vi "npks.vi"() -> ()   [LabVIEW 2015]
uses:
  <vilib>/LabVIEW Open Source Project/MQTT Control Packets/Control Packets/SUBACK/Subscription Success Code.ctl
  <vilib>/LabVIEW Open Source Project/MQTT Control Packets/Control Packets/ControlPacket/QualityOfService -- enum.ctl
  <vilib>/LabVIEW Open Source Project/MQTT Control Packets/Control Packets/SUBSCRIBE/Topic Subscription -- cluster.ctl
  <vilib>/LabVIEW Open Source Project/MQTT Control Packets/Control Packets/CONNECT/ConnectFlags -- cluster.ctl
  <vilib>/LabVIEW Open Source Project/MQTT Client/Client class/Client.lvclass/Client.ctl
  <vilib>/LabVIEW Open Source Project/MQTT Connection/MQTT_Base/Base Class/MQTT_Base.lvclass/MQTT_Base.ctl
  <vilib>/LabVIEW Open Source Project/MQTT Control Packets/Control Packets/ControlPacket/ControlPacket.lvclass/ControlPacket.ctl
  <vilib>/Modbus/master/Create Master Instance (Serial).vi
  <vilib>/LabVIEW Open Source Project/MQTT Control Packets/Control Packets/PUBLISH/PUBLISH.lvclass
  <vilib>/Modbus/master/Modbus Master.lvclass
  <vilib>/LabVIEW Open Source Project/MQTT Client/Client class/Client.lvclass
  <vilib>/LabVIEW Open Source Project/MQTT Connection/MQTT_Base/Base Class/MQTT_Base.lvclass
  <vilib>/LabVIEW Open Source Project/MQTT Control Packets/Control Packets/ControlPacket/ControlPacket.lvclass
  <vilib>/LabVIEW Open Source Project/Connection/Connection.TCP/Connection.TCP.lvclass
  <vilib>/LabVIEW Open Source Project/Connection/Connection.LocalQueue/Connection.LocalQueue.lvclass
  <vilib>/LabVIEW Open Source Project/Connection/Connection/Connection.lvclass
  <vilib>/LabVIEW Open Source Project/MQTT Control Packets/Control Packets/SUBACK/SUBACK.lvclass
  <vilib>/LabVIEW Open Source Project/MQTT Control Packets/Control Packets/SUBSCRIBE/SUBSCRIBE.lvclass
  <vilib>/LabVIEW Open Source Project/MQTT Control Packets/Control Packets/CONNECT/CONNECT.lvclass
panel:
  out "K":bool
  in  "Payload":T1={"Will Topic"="", "Will Message"="", "Username"="jCpxJWfzRMyJc3yBgeDZF8tX4bProa3f", "Password"="dyi3Gar4LryWnGSwkNjPS2jYQKdPeLnd"}
  in  "Will Message":string
  in  "Will Topic":string
  out "N":bool
  out "P":bool
  in  "SET POINT N":dbl=300.0
  in  "SET POINT K":dbl=20.0
  in  "holding register value K":u16
  in  "SET POINT P":dbl=300.0
  in  "holding register value P":u16
  out "error out 9":errorcluster
  out "K":string="                        199"
  out "Type 3":variant
  out "Topic 3":string
  out "error out 8":cluster{}
  out "Suback":bool
  out "source 2":string
  out "code":i32
  out "status":bool
  out "source":string
  in  "error in (no error)":errorcluster
  in  "ID (empty:generate new)":string="e22b6e7b-a166-44ae-bd9e-56b8868e9341"
  in  "Connect Flags":T2={"Reserved"=FALSE, "Clean Session"=TRUE, "Will Flag"=FALSE, "Will QoS 1"=FALSE, "Will QoS 2"=FALSE, "Will Retain"=FALSE, "Password Flag"=TRUE, "User Name Flag"=TRUE}
  out "error out 7":errorcluster
  out "error out 2":errorcluster
  out "Incoming Message":u8[](array[numeric]) format="%08b"
  out "error out 6":errorcluster
  out "P":string
  out "Type 2":variant
  out "Topic 2":string
  out "error out 5":cluster{}
  out "error out 4":errorcluster
  out "N":string
  out "Type":variant
  out "Topic":string
  out "error out 3":cluster{"status":bool, "code":i32}
  in  "Subscribe":bool
  in  "Topic Subscriptions":T3[](array[typedef])=[{"Topic Filter"="@msg/D1/LED1", "QoS"=enum."0 (At Most Once)"}, {"Topic Filter"="@msg/D1/LED2", "QoS"=enum."0 (At Most Once)"}, {"Topic Filter"="@msg/D1/LED3", "QoS"=enum."0 (At Most Once)"}]
  out "Subscription Success":T5[](array[typedef])
  out "Published":bool
  out "number (0 to 1)":dbl
  in  "Publish":bool
  in  "Stop Client":bool
  out "Numeric":i32
  out "element":u16
  out "Gauge":dbl(knob) scale=0.0..500.0
  in  "Knob Set Speed":i32(knob) scale=0.0..100.0
  in  "address":u16=100
  in  "holding register value N":u16
  in  "Write Button":bool
  in  "baud rate (9600)":u32=9600
  in  "flow control (None)":u16(ring) items=["None", "XON/XOFF", "RTS/CTS", "XON/XOFF & RTS/CTS", "DTR/DSR", "XON/XOFF & DTR/DSR"]
  in  "parity (Even)":u16(ring) items=["None", "Odd", "Even"]
  in  "unit ID":u8=10
  out "error out":errorcluster
  out "register values":u16[](array[numeric])
  in  "number of input registers":u16=10
  in  "starting address":u16=100
  in  "stop":bool
  in  "serial type":enum16{"RTU", "ASCII"}(ring)
  in  "VISA resource name":refnum<visa-resource-name>
  # "Setting"
  # "Connect Netpie"
  # "Set Point"
  # "Status"
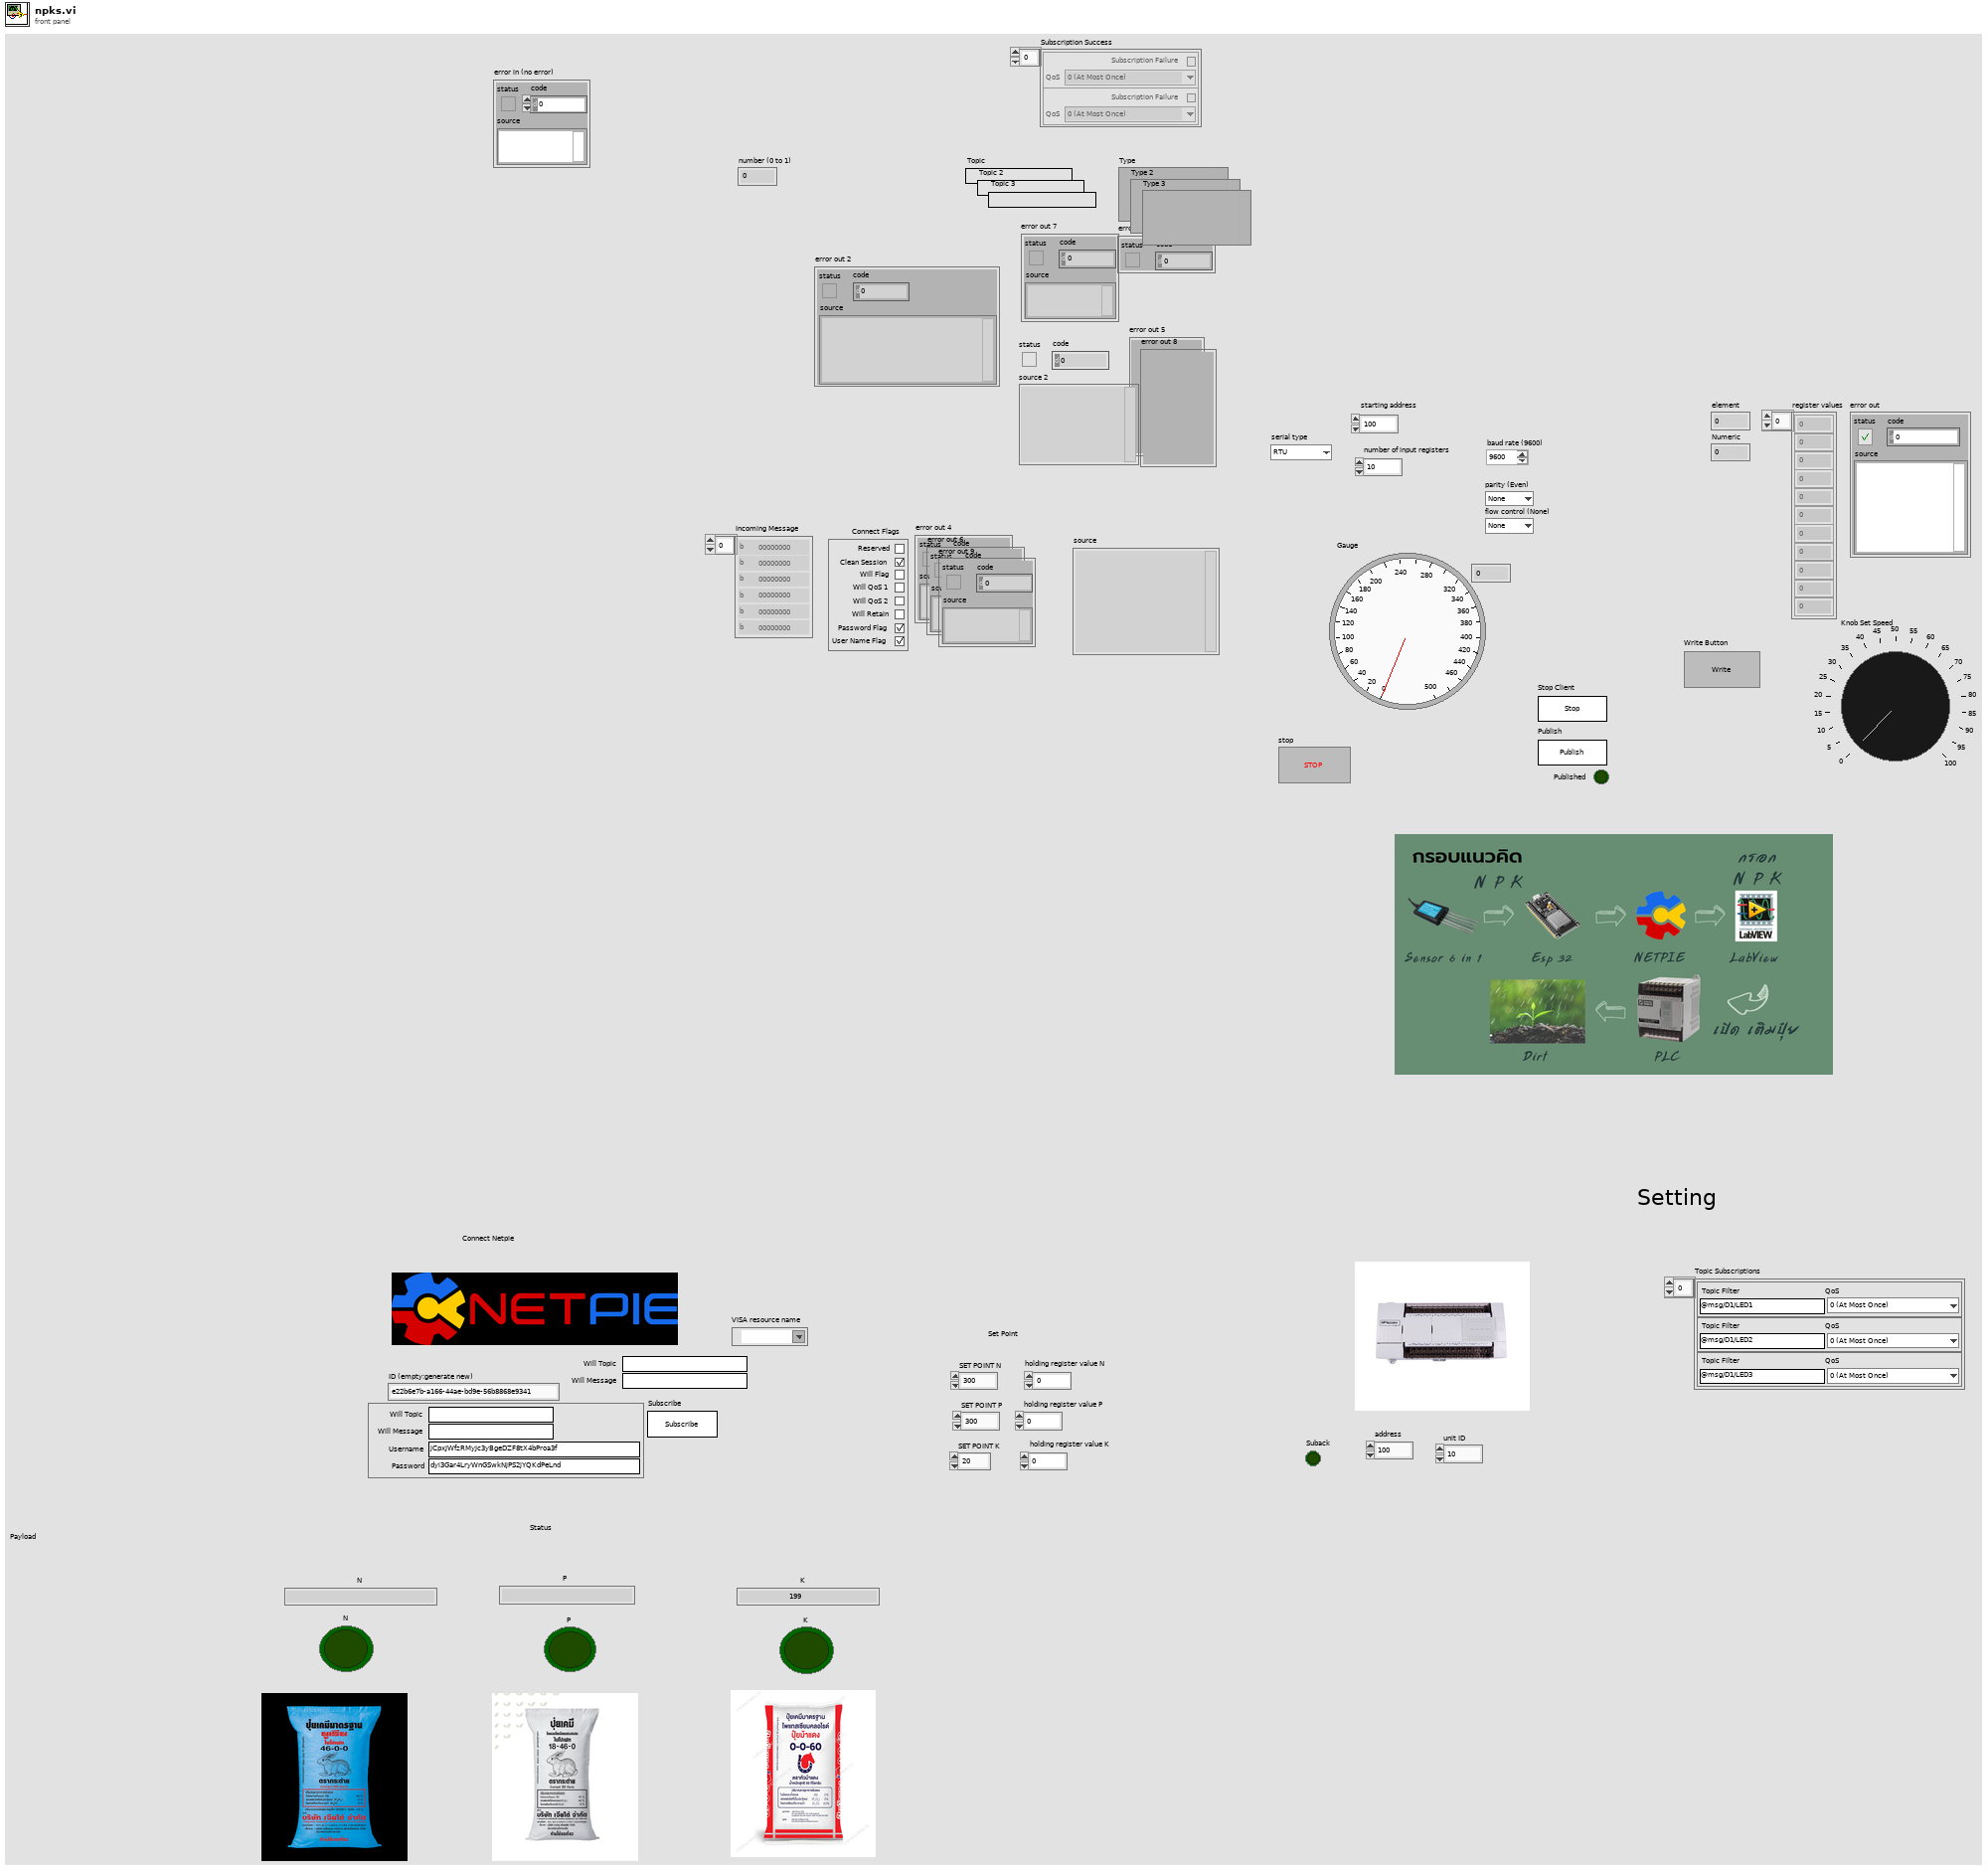
[diagram p1: front panel]
types:
  T1 = cluster{"Will Topic":string, "Will Message":string, "Username":string, "Password":string}
  T2 = typedef "MQTT_Control_Packets.lvlib/CONNECT.lvclass/ConnectFlags -- cluster.ctl" = cluster{"Reserved":bool, "Clean Session":bool, "Will Flag":bool, "Will QoS 1":bool, "Will QoS 2":bool, "Will Retain":bool, "Password Flag":bool, "User Name Flag":bool}
  T3 = typedef "MQTT_Control_Packets.lvlib/SUBSCRIBE.lvclass/Topic Subscription -- cluster.ctl" = cluster{"Topic Filter":string, "QoS":T4}
  T4 = typedef "MQTT_Control_Packets.lvlib/ControlPacket.lvclass/QualityOfService -- enum.ctl" = enum16{"0 (At Most Once)", "1 (At Least Once)", "2 (Exactly Once)"}
  T5 = typedef "MQTT_Control_Packets.lvlib/SUBACK.lvclass/Subscription Success Code.ctl" = cluster{"Subscription Failure":bool, "QoS":T4}
  T6 = typedef "MQTT Client.lvlib/Client.lvclass/Public Events -- cluster.ctl" = cluster{"Connection Status":refnum<user-event>, "Connected":refnum<user-event>, "Application Message":refnum<user-event>}
  T7 = typedef "MQTT Base.lvlib/MQTT_Base.lvclass/Public Events -- cluster.ctl" = cluster{"Stop Event":refnum<user-event>, "Error Event":refnum<user-event>, "Inbound Message":refnum<user-event>}
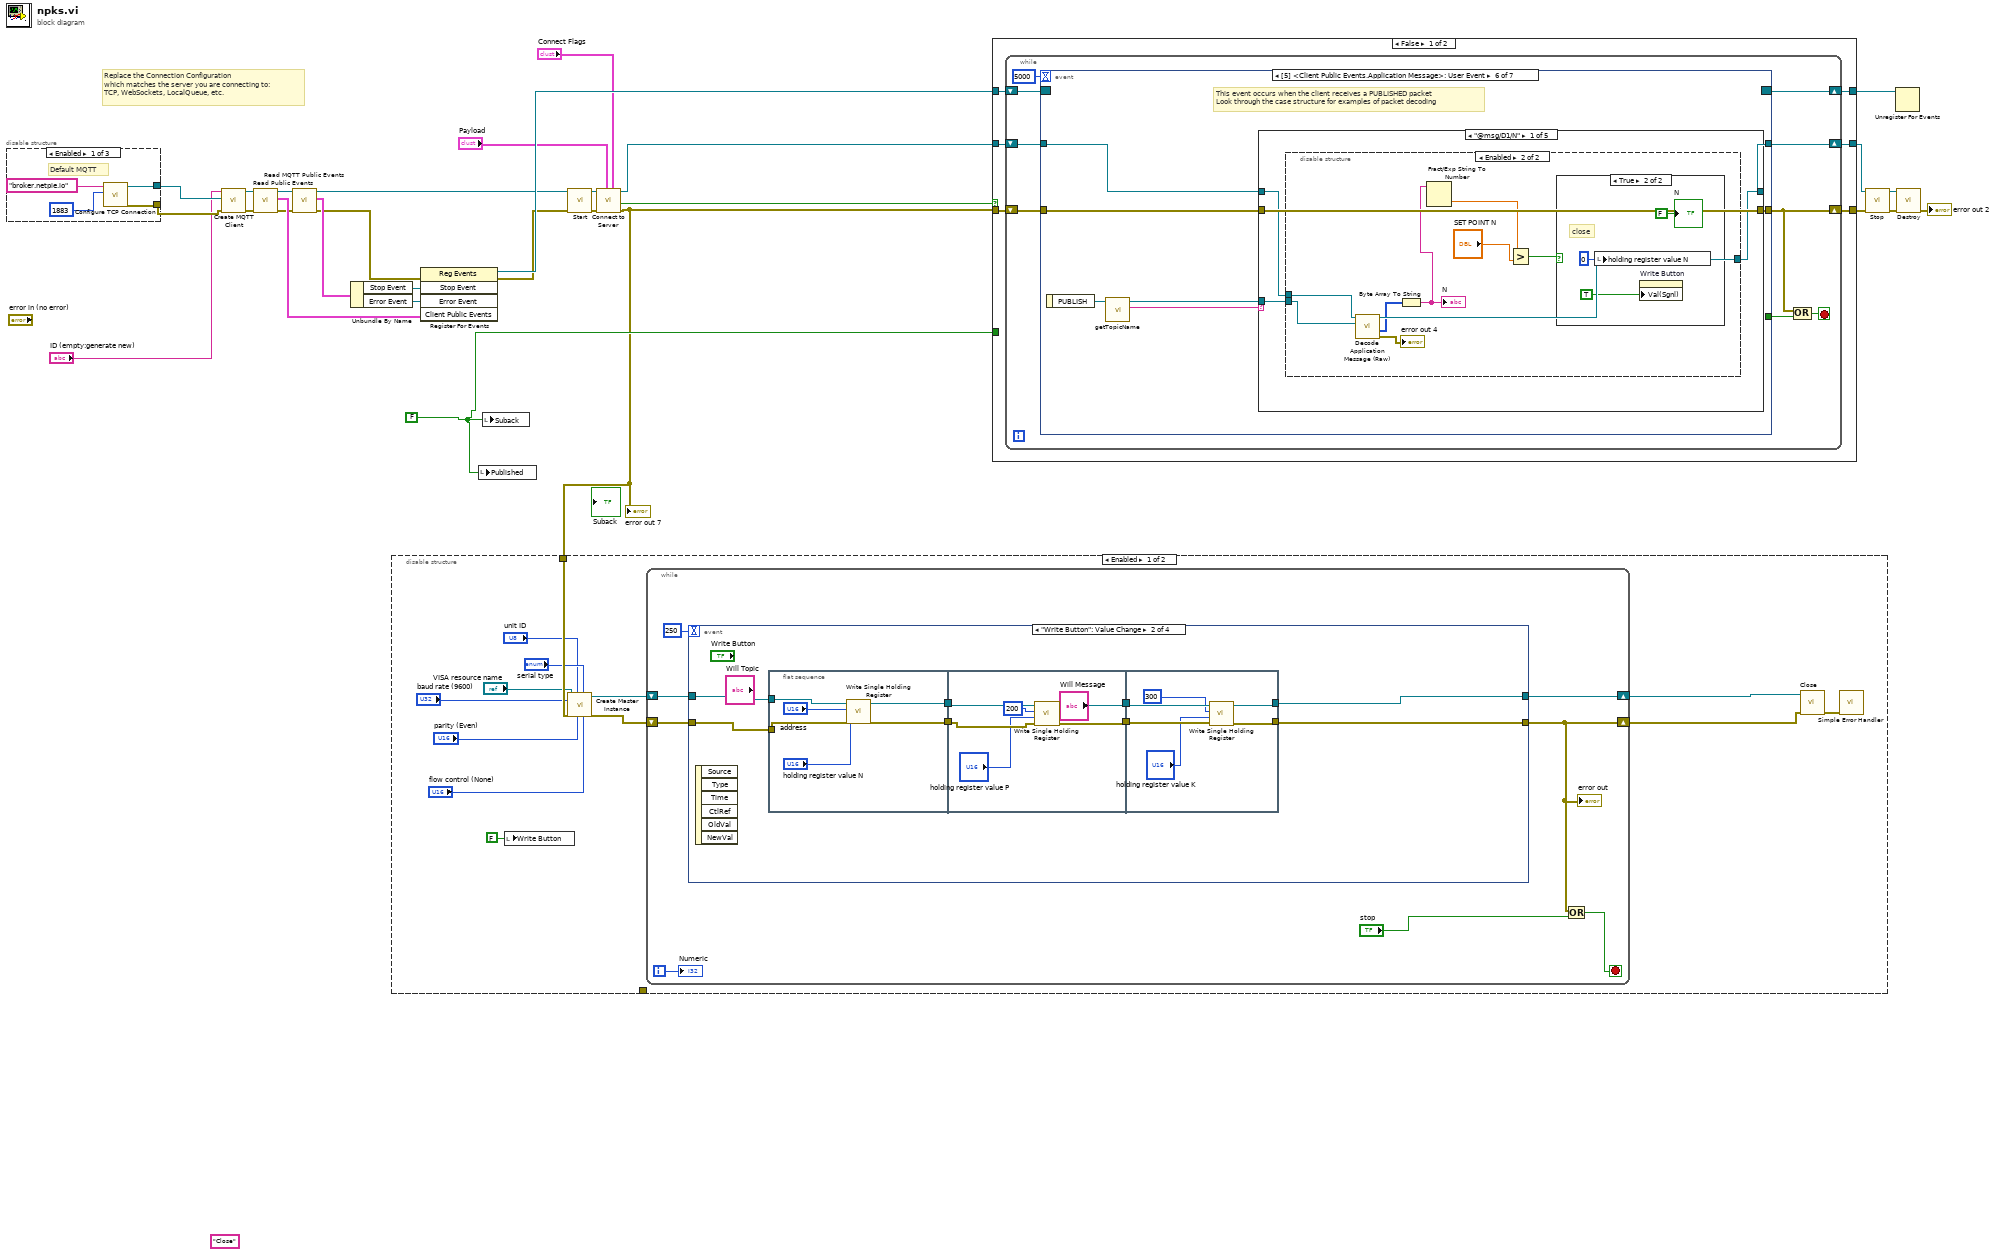
[diagram p0: block diagram]
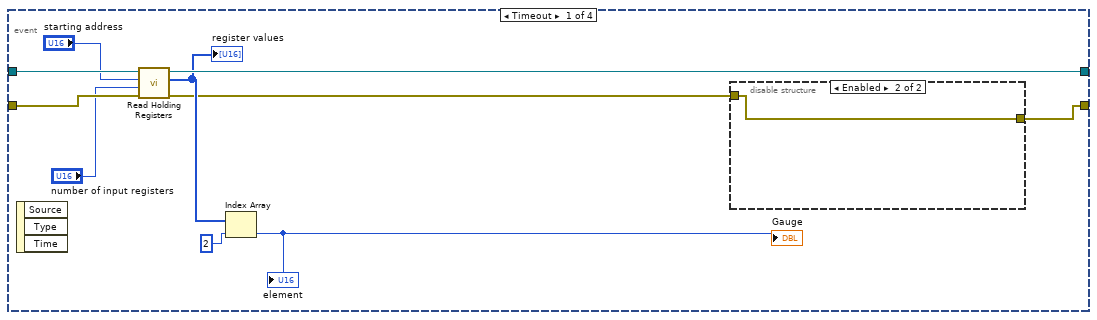
[diagram p2: hidden frame]
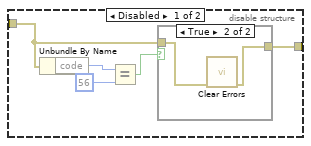
[diagram p3: hidden frame]
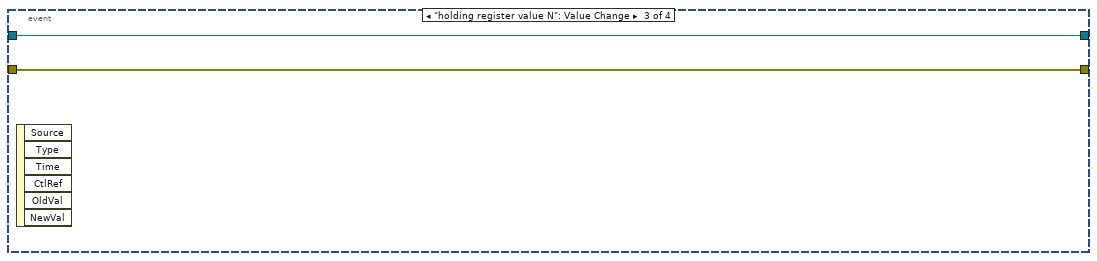
[diagram p5: hidden frame]
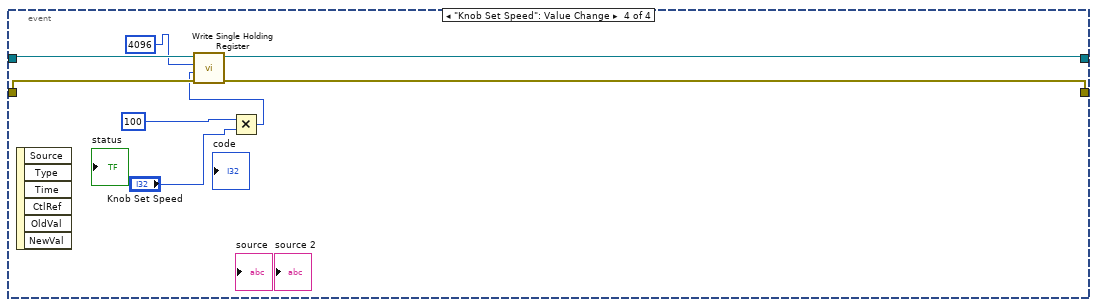
[diagram p6: hidden frame]
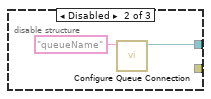
[diagram p8: hidden frame]
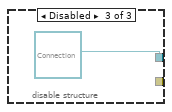
[diagram p9: hidden frame]
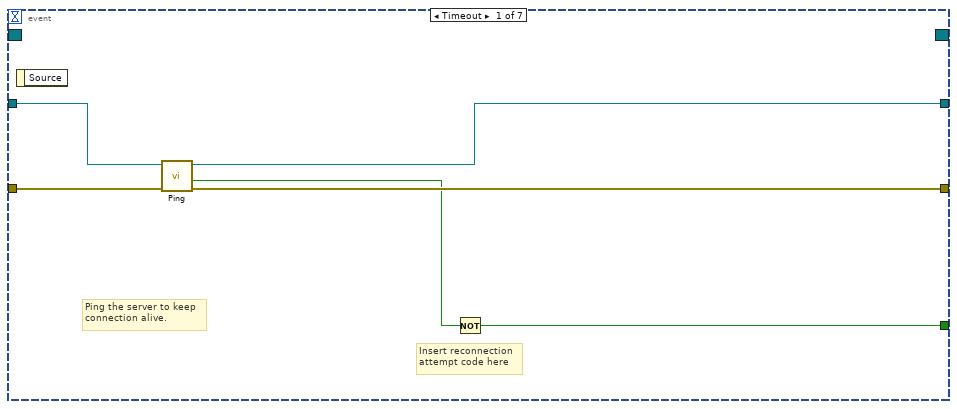
[diagram p10: hidden frame]
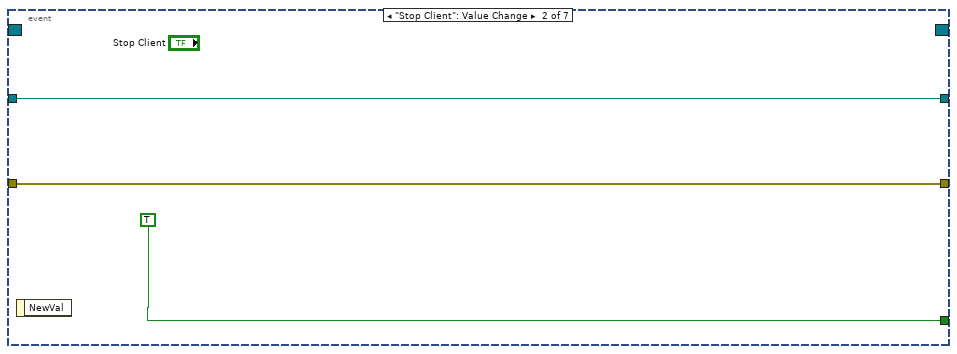
[diagram p11: hidden frame]
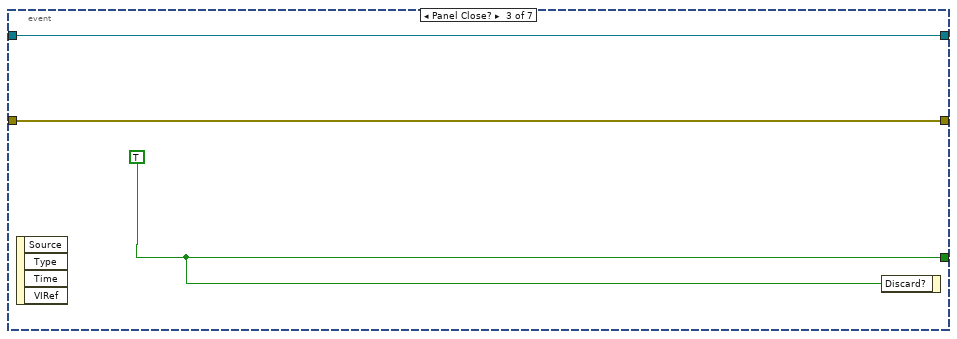
[diagram p12: hidden frame]
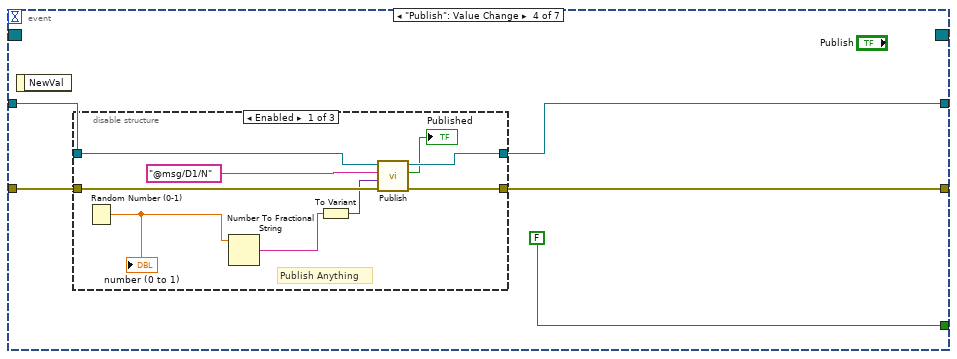
[diagram p13: hidden frame]
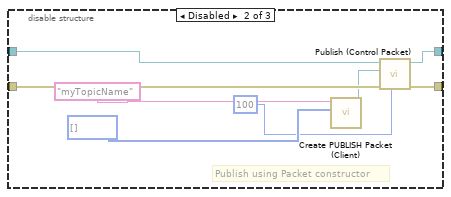
[diagram p14: hidden frame]
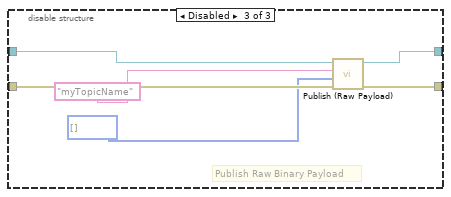
[diagram p15: hidden frame]
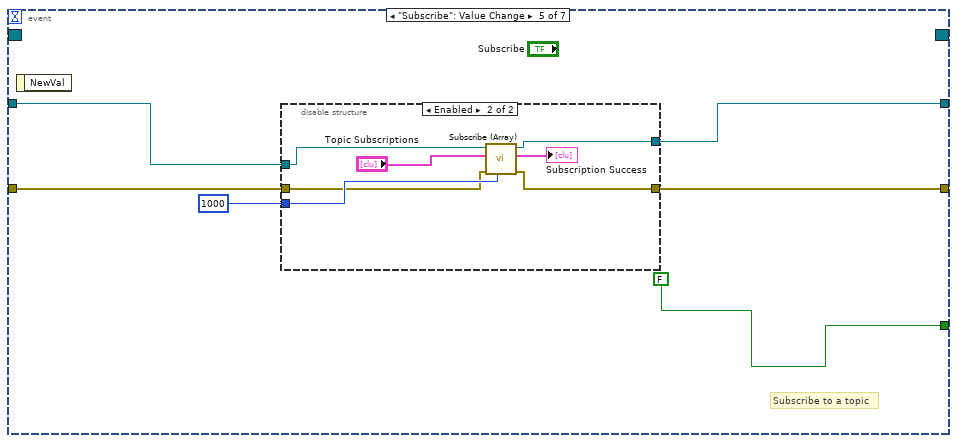
[diagram p16: hidden frame]
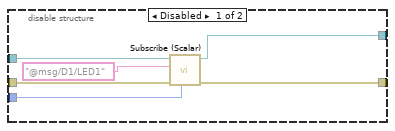
[diagram p17: hidden frame]
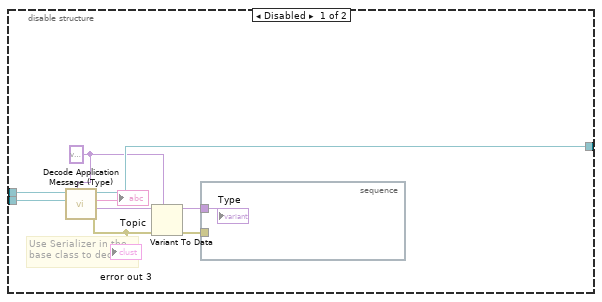
[diagram p18: hidden frame]
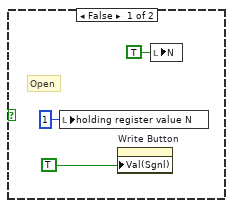
[diagram p19: hidden frame]
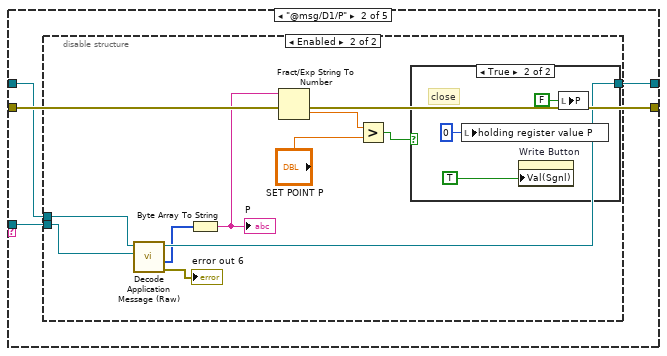
[diagram p20: hidden frame]
diagram:
  (unwired) "Close"
  w3 = FALSE ("Suback")
  # "Replace the Connection Configuration\nwhich matches the server you are connecting to:\nTCP, WebSockets, LocalQueue, etc."
  n1 = disable-structure shown="Enabled" {
    disable-tunnel: [w32 w35 refnum<class "Connection.lvclass"> refnum ("Connection Configuration")] -> w29
    disable-tunnel: [w30 _ _] -> w6
    frame Enabled {
      # "Default MQTT"
      n2 = call <vilib>:"Configure TCP Connection.vi"("remote port (80)"=u16 1883, "address (localhost)"="broker.netpie.io") -> ("error out"=w30:errorcluster, "Connection.TCP"=w32:refnum<class "Connection.TCP.lvclass">)  [unwired: 8 in]
    }
    frame Disabled {
      n3 = call <vilib>:"Configure Queue Connection.vi"("Queue Name"="queueName") -> ("Connection.LocalQueue"=w35:refnum<class "Connection.LocalQueue.lvclass">)  [unwired: 9 in, 1 out]
    }
    frame Disabled {
    }
  }
  n4 = call <vilib>:"Create MQTT Client.vi"("error in (no error)"=w6, "Connection Configuration"=w29, "ID (empty:generate new)"="ID (empty:generate new)") -> ("error out"=w9:errorcluster, "Client out"=w7:refnum<class "Client.lvclass">)  [unwired: 7 in]
  n5 = call <vilib>:"Read Public Events.vi"("error in (no error)"=w9, "Client in"=w7) -> ("error out"=w10:errorcluster, "Client Public Events"=w12:T6, "Client out"=w8:refnum<class "Client.lvclass">)  [unwired: 7 in]
  n6 = call <vilib>:"Read MQTT Public Events.vi"("error in (no error)"=w10, "MQTT_Base in"=w8) -> ("error out"=w11:errorcluster, "MQTT Public Events"=w23:T7, "MQTT_Base out"=w14:refnum<class "Client.lvclass">)  [unwired: 7 in]
  n7 = Unbundle By Name(w23) -> ("Stop Event"=w21:refnum<user-event>, "Error Event"=w22:refnum<user-event>)
  n8 = register-events(error in=w11, w21, w22, w12) -> (reference out=w17:refnum<event-registration>, error out=w13:errorcluster)  [unwired: 1 in]
  n9 = local write "Published"(w3) -> ()
  n10 = local write "Suback"(w3) -> ()
  n11 = call <vilib>:"Start.vi"("error in (no error)"=w13, "MQTT_Base in"=w14) -> ("error out"=w16:errorcluster, "MQTT_Base out"=w15:refnum<class "Client.lvclass">)  [unwired: 7 in, 1 out]
  n12 = call <vilib>:"Connect to Server.vi"("Connect Flags"="Connect Flags", "Payload"="Payload", "error in (no error)"=w16, "Client in"=w15) -> ("error out"=w2:errorcluster, "timed out"=w19:bool, "Client out"=w20:refnum<class "Client.lvclass">)  [unwired: 4 in, 1 out]
  "error out 7" <- w2
  n13 = disable-structure shown="Enabled" {
    disable-tunnel: w2 -> [w49 w113]
    disable-tunnel: [_ w113] -> _
    frame Enabled {
      n14 = local write "Write Button"(FALSE ("Write Button")) -> ()
      n15 = call-poly <vilib>:"Create Master Instance.vi"("flow control (None)"="flow control (None)", "serial type"="serial type", "parity (Even)"="parity (Even)", "unit ID"="unit ID", "error in (no error)"=w49, "baud rate (9600)"="baud rate (9600)", "VISA resource name"="VISA resource name") -> ("error out"=w48:errorcluster, "serial master instance"=w45:refnum<class "Modbus Master.lvclass">)  [unwired: 3 in]
      n16 = while {
        shift-right: [w54] -> w42
        shift-left: w45 -> [w57]
        shift-right: [w53] -> w43
        shift-left: w48 -> [w56]
        i -> [w50]
        stop <- w55 stop-if-true
        n17 = event shown="[1] \"Write Button\": Value Change" {
          selector: _ -> [_ _ _ _]
          dyn-events: _ -> [_ _ _ _]
          timeout: 250 -> [_ _ _ _]
          tunnel: w57 -> [w67 w84 w104 w112]
          tunnel: w56 -> [w66 w83 w103 w110]
          tunnel: [w65 w82 w104 w111] -> w54
          tunnel: [w58 w81 w103 w109] -> w53
          event Timeout {
            n18 = event-data() -> ()  [unwired: 1 in, 3 out]
            n19 = call-dynamic "Read Holding Registers.vi"("error in (no error)"=w66, "number of holding registers"="number of input registers", "starting address"="starting address", "Modbus master in"=w67) -> ("error out"=w59:errorcluster, "register values"=w62:u16[], "Modbus master out"=w65:refnum<class "Modbus Master.lvclass">)  [unwired: 5 in]
            "register values" <- w62
            n20 = Index Array(array=w62, index=2) -> (element=→"Gauge" →"element":u16)
            n21 = disable-structure shown="Enabled" {
              disable-tunnel: w59 -> [w69 w76]
              disable-tunnel: [w68 w76] -> w58
              frame Disabled {
                n22 = Unbundle By Name(w69) -> ("code"=w72:i32)
                n23 = Equal?(x=w72, y=56) -> (x = y?=w70:bool)
                n24 = case shown="True" w70 {
                  tunnel: w69 -> [w73 w75]
                  tunnel: [w73 w74] -> w68
                  frame False {
                  }
                  frame True {
                    n25 = call <vilib>:"Clear Errors.vi"("error in (no error)"=w75) -> ("error out"=w74:errorcluster)  [unwired: 5 in, 1 out]
                  }
                }
              }
              frame Enabled {
              }
            }
          }
          event "Write Button": Value Change {
            n26 = event-data() -> ()  [unwired: 1 in, 6 out]
            n27 = flat-sequence {
              tunnel: w84 -> [w90]
              tunnel: w83 -> [w89]
              tunnel: [w88] -> w80
              tunnel: [w87] -> w79
              tunnel: w80 -> [w95]
              tunnel: w79 -> [w96]
              tunnel: [w94] -> w78
              tunnel: [w93] -> w77
              tunnel: [w99] -> w81
              tunnel: [w101] -> w82
              tunnel: w78 -> [w102]
              tunnel: w77 -> [w100]
              frame #0 {
                n28 = call-dynamic "Write Single Holding Register.vi"("error in (no error)"=w89, "holding register value"="holding register value N", "address"="address", "Modbus master in"=w90) -> ("error out"=w87:errorcluster, "Modbus master out"=w88:refnum<class "Modbus Master.lvclass">)  [unwired: 6 in]
              }
              frame #1 {
                n29 = call-dynamic "Write Single Holding Register.vi"("error in (no error)"=w96, "holding register value"="holding register value P", "address"=u16 200, "Modbus master in"=w95) -> ("error out"=w93:errorcluster, "Modbus master out"=w94:refnum<class "Modbus Master.lvclass">)  [unwired: 6 in]
              }
              frame #2 {
                n30 = call-dynamic "Write Single Holding Register.vi"("error in (no error)"=w100, "holding register value"="holding register value K", "address"=u16 300, "Modbus master in"=w102) -> ("error out"=w99:errorcluster, "Modbus master out"=w101:refnum<class "Modbus Master.lvclass">)  [unwired: 6 in]
              }
            }
          }
          event "holding register value N": Value Change {
            n31 = event-data() -> ()  [unwired: 1 in, 6 out]
          }
          event "Knob Set Speed": Value Change {
            n32 = event-data() -> ()  [unwired: 1 in, 6 out]
            n33 = Multiply(x=100, y="Knob Set Speed") -> (x*y=w106:i32)
            n34 = call-dynamic "Write Single Holding Register.vi"("error in (no error)"=w110, "holding register value"=w106, "address"=u16 4096, "Modbus master in"=w112) -> ("error out"=w109:errorcluster, "Modbus master out"=w111:refnum<class "Modbus Master.lvclass">)  [unwired: 6 in]
          }
        }
        "error out" <- w53
        n35 = Or(x=w53, y="stop") -> (x .or. y?=w55:bool)
        "Numeric" <- w50
      }
      n36 = call-dynamic "Close.vi"("error in (no error)"=w43, "Modbus master in"=w42) -> ("error out"=w41:errorcluster)  [unwired: 9 in]
      n37 = call <vilib>:"Simple Error Handler.vi"("error in (no error)"=w41) -> ()  [unwired: 4 in, 5 out]
    }
    frame Disabled {
    }
  }
  n38 = case shown="False" w19 {
    tunnel: w17 -> [w119 w299]
    tunnel: [w118 w299] -> w18
    tunnel: w2 -> [w115 w297]
    tunnel: w20 -> [w117 w298]
    tunnel: [w116 w298] -> w25
    tunnel: [w114 w297] -> w27
    tunnel: w3 -> [_ _]
    frame False {
      n39 = while {
        shift-right: [w127] -> w118
        shift-left: w119 -> [w128]
        shift-right: [w120] -> w116
        shift-left: w117 -> [w121]
        shift-right: [w125] -> w114
        shift-left: w115 -> [w126]
        stop <- w124 stop-if-true
        n40 = event shown="[5] <Client Public Events.Application Message>: User Event" {
          selector: w128 -> [_ _ _ _ _ _ _]
          dyn-events: [_ _ _ _ _ _ _] -> w127
          timeout: 5000 -> [_ _ _ _ _ _ _]
          tunnel: w126 -> [w133 w136 w138 w143 w172 w190 w296]
          tunnel: [w131 w136 w138 w142 w171 w191 w296] -> w125
          tunnel: [w130 TRUE w140 FALSE FALSE _ TRUE] -> w123
          tunnel: w121 -> [w134 w137 w139 w144 w173 w193 w294]
          tunnel: [w132 w137 w139 w141 w170 w192 w294] -> w120
          event Timeout {
            # "Insert reconnection\nattempt code here"
            # "Ping the server to keep\nconnection alive."
            n41 = event-data() -> ()  [unwired: 1 in, 1 out]
            n42 = call <vilib>:"Ping.vi"("error in (no error)"=w133, "Client in"=w134) -> ("error out"=w131:errorcluster, "Server responded"=w129:bool, "Client out"=w132:refnum<class "Client.lvclass">)  [unwired: 6 in, 1 out]
            n43 = Not(x=w129) -> (.not. x?=w130:bool)
          }
          event "Stop Client": Value Change {
            n44 = event-data() -> ()  [unwired: 1 in, 1 out]
          }
          event Panel Close? {
            w140 = TRUE
            n45 = event-data() -> ()  [unwired: 1 in, 4 out]
            n46 = event-data("Discard?"=w140) -> ()  [unwired: 1 in, 1 out]
          }
          event "Publish": Value Change {
            n47 = event-data() -> ()  [unwired: 1 in, 1 out]
            n48 = disable-structure shown="Enabled" {
              disable-tunnel: w144 -> [w154 w160 w168]
              disable-tunnel: w143 -> [w153 w158 w165]
              disable-tunnel: [w152 w157 w166] -> w142
              disable-tunnel: [w151 w159 w167] -> w141
              frame Enabled {
                # "Publish Anything"
                n49 = Random Number (0-1)() -> (number: 0 to 1=w147:dbl)
                "number (0 to 1)" <- w147
                n50 = Number To Fractional String(number=w147) -> (F-format string=w146:string)  [unwired: 3 in]
                n51 = To Variant(anything=w146) -> (Variant=w149:variant)
                n52 = call <vilib>:"Publish.vi"("error in (no error)"=w153, "Payload"=w149, "Topic Name (empty: Payload name)"="@msg/D1/N", "Client in"=w154) -> ("error out"=w152:errorcluster, "Published"=→"Published":bool, "Client out"=w151:refnum<class "Client.lvclass">)  [unwired: 5 in]
              }
              frame Disabled {
                # "Publish using Packet constructor"
                n53 = call <vilib>:"Create PUBLISH Packet (Client).vi"("Payload"=u8[] [], "Topic Name"="myTopicName" ("Topic Name (empty: Payload name)")) -> ("PUBLISH"=w155:refnum<class "PUBLISH.lvclass">)  [unwired: 6 in, 3 out]
                n54 = call <vilib>:"Publish (Control Packet).vi"("timeout (1000ms)"=100 ("timeout (0ms : no ack)"), "error in (no error)"=w158, "PUBLISH"=w155, "Client in"=w160) -> ("error out"=w157:errorcluster, "Client out"=w159:refnum<class "Client.lvclass">)  [unwired: 5 in, 1 out]
              }
              frame Disabled {
                # "Publish Raw Binary Payload"
                n55 = call <vilib>:"Publish (Raw Payload).vi"("error in (no error)"=w165, "Binary Payload"=u8[] [] ("Payload"), "Topic Name"="myTopicName" ("Topic Name (empty: Payload name)"), "Client in"=w168) -> ("error out"=w166:errorcluster, "Client out"=w167:refnum<class "Client.lvclass">)  [unwired: 5 in, 1 out]
              }
            }
          }
          event "Subscribe": Value Change {
            # "Subscribe to a topic"
            n56 = event-data() -> ()  [unwired: 1 in, 1 out]
            n57 = disable-structure shown="Enabled" {
              disable-tunnel: w173 -> [w181 w188]
              disable-tunnel: w172 -> [w179 w184]
              disable-tunnel: [w178 w183] -> w171
              disable-tunnel: [w177 w185] -> w170
              disable-tunnel: 1000 ("timeout (100ms)") -> [w175 w187]
              frame Disabled {
                n58 = call <vilib>:"Subscribe (Scalar).vi"("timeout (1000ms)"=w175, "error in (no error)"=w179, "Topic Filter"="@msg/D1/LED1" ("Topic Name (empty: Payload name)"), "Client in"=w181) -> ("error out"=w178:errorcluster, "Ack"=w176:bool, "Client out"=w177:refnum<class "Client.lvclass">)  [unwired: 5 in]
              }
              frame Enabled {
                n59 = call <vilib>:"Subscribe (Array).vi"("timeout (1000ms)"=w187, "error in (no error)"=w184, "Topic Subscriptions"="Topic Subscriptions", "Client in"=w188) -> ("error out"=w183:errorcluster, "Subscription Success"=→"Subscription Success":T5[], "Client out"=w185:refnum<class "Client.lvclass">)  [unwired: 5 in]
              }
            }
          }
          event User Event {
            # "This event occurs when the client receives a PUBLISHED packet\nLook through the case structure for examples of packet decoding"
            n60 = event-data() -> ("PUBLISH"=w195:refnum<class "PUBLISH.lvclass">)  [unwired: 1 in]
            n61 = call <vilib>:"getTopicName.vi"("PUBLISH in"=w195) -> ("Topic"=w194:string, "PUBLISH out"=w189:refnum<class "PUBLISH.lvclass">)  [unwired: 8 in, 1 out]
            n62 = case shown="\"@msg/D1/N\"" w194 {
              tunnel: w193 -> [w198 w227 w257 w289 w293]
              tunnel: [w197 w226 w254 w288 w293] -> w192
              tunnel: [w199 w228 w258 w286 w292] -> w191
              tunnel: w190 -> [w199 w228 w258 w285 w292]
              tunnel: w189 -> [w196 w225 w256 w284 w291]
              frame "@msg/D1/N" {
                n63 = disable-structure shown="Enabled" {
                  disable-tunnel: w198 -> [w206 w218]
                  disable-tunnel: [w205 w216] -> w197
                  disable-tunnel: w196 -> [w204 w217]
                  frame Disabled {
                    w202 = variant ("Type")
                    # "Use Serializer in the\nbase class to decode"
                    n64 = call <vilib>:"Decode Application Message (Type).vi"("Type"=w202, "PUBLISH"=w204, "Client in"=w206) -> ("error out"=w201:errorcluster, "Payload"=w203:variant, "Topic"=→"Topic":string, "Client out"=w205:refnum<class "Client.lvclass">)  [unwired: 5 in]
                    "error out 3" <- w201
                    n65 = Variant To Data(error in=w201, type=w202, Variant=w203) -> (data=w208:variant, error out=w207:errorcluster)
                    n66 = stacked-sequence {
                      tunnel: w208 -> [w209]
                      tunnel: w207 -> [_]
                      frame #0 {
                        "Type" <- w209
                      }
                    }
                  }
                  frame Enabled {
                    n67 = call <vilib>:"Decode Application Message (Raw).vi"("PUBLISH"=w217, "Client in"=w218) -> ("error out"=→"error out 4":errorcluster, "Payload"=w214:u8[], "Client out"=w216:refnum<class "Client.lvclass">)  [unwired: 6 in, 1 out]
                    n68 = Byte Array To String(unsigned byte array=w214) -> (string=w212:string)
                    "N" <- w212
                    n69 = Fract/Exp String To Number(string=w212) -> (number=w210:dbl)  [unwired: 3 in, 1 out]
                    n70 = Greater?(x=w210, y="SET POINT N") -> (0:w213:bool)
                    n71 = case shown="True" w213 {
                      frame False {
                        # "Open"
                        n72 = local write "holding register value N"(u16 1 ("holding register value P")) -> ()
                        n73 = property on="Write Button" class="Bool (strict)"("Val(Sgnl)"=TRUE ("Value (Signaling)")) -> ()  [unwired: 2 in, 2 out]
                        n74 = local write "N"(TRUE ("N")) -> ()
                      }
                      frame True {
                        # "close"
                        n75 = local write "holding register value N"(u16 0 ("holding register value P")) -> ()
                        n76 = property on="Write Button" class="Bool (strict)"("Val(Sgnl)"=TRUE ("Value (Signaling)")) -> ()  [unwired: 2 in, 2 out]
                        "N" <- FALSE
                      }
                    }
                  }
                }
              }
              frame "@msg/D1/P" {
                n77 = disable-structure shown="Enabled" {
                  disable-tunnel: w227 -> [w235 w247]
                  disable-tunnel: [w234 w245] -> w226
                  disable-tunnel: w225 -> [w233 w246]
                  frame Disabled {
                    w231 = variant ("Type")
                    # "Use Serializer in the\nbase class to decode"
                    n78 = call <vilib>:"Decode Application Message (Type).vi"("Type"=w231, "PUBLISH"=w233, "Client in"=w235) -> ("error out"=w230:errorcluster, "Payload"=w232:variant, "Topic"=→"Topic 2":string, "Client out"=w234:refnum<class "Client.lvclass">)  [unwired: 5 in]
                    "error out 5" <- w230
                    n79 = Variant To Data(error in=w230, type=w231, Variant=w232) -> (data=w237:variant, error out=w236:errorcluster)
                    n80 = stacked-sequence {
                      tunnel: w237 -> [w238]
                      tunnel: w236 -> [_]
                      frame #0 {
                        "Type 2" <- w238
                      }
                    }
                  }
                  frame Enabled {
                    n81 = call <vilib>:"Decode Application Message (Raw).vi"("PUBLISH"=w246, "Client in"=w247) -> ("error out"=→"error out 6":errorcluster, "Payload"=w243:u8[], "Client out"=w245:refnum<class "Client.lvclass">)  [unwired: 6 in, 1 out]
                    n82 = Byte Array To String(unsigned byte array=w243) -> (string=w242:string)
                    "P" <- w242
                    n83 = Fract/Exp String To Number(string=w242) -> (number=w241:dbl)  [unwired: 3 in, 1 out]
                    n84 = Greater?(x=w241, y="SET POINT P") -> (0:w239:bool)
                    n85 = case shown="True" w239 {
                      frame False {
                        # "Open"
                        n86 = local write "holding register value P"(u16 1 ("holding register value P")) -> ()
                        n87 = property on="Write Button" class="Bool (strict)"("Val(Sgnl)"=TRUE ("Value (Signaling)")) -> ()  [unwired: 2 in, 2 out]
                        "P" <- TRUE ("P")
                      }
                      frame True {
                        # "close"
                        n88 = local write "holding register value P"(u16 0 ("holding register value P")) -> ()
                        n89 = property on="Write Button" class="Bool (strict)"("Val(Sgnl)"=TRUE ("Value (Signaling)")) -> ()  [unwired: 2 in, 2 out]
                        n90 = local write "P"(FALSE ("P")) -> ()
                      }
                    }
                  }
                }
              }
              frame "@msg/D1/K" {
                n91 = feedback #1() -> (w254:refnum<class "Client.lvclass">)  [unwired: 1 in]
                n92 = disable-structure shown="Enabled" {
                  disable-tunnel: w257 -> [w265 w277]
                  disable-tunnel: [w264 w275] -> w255
                  disable-tunnel: w256 -> [w263 w276]
                  disable-tunnel: w254 -> [_ _]
                  frame Disabled {
                    w261 = variant ("Type")
                    # "Use Serializer in the\nbase class to decode"
                    n93 = call <vilib>:"Decode Application Message (Type).vi"("Type"=w261, "PUBLISH"=w263, "Client in"=w265) -> ("error out"=w260:errorcluster, "Payload"=w262:variant, "Topic"=→"Topic 3":string, "Client out"=w264:refnum<class "Client.lvclass">)  [unwired: 5 in]
                    "error out 8" <- w260
                    n94 = Variant To Data(error in=w260, type=w261, Variant=w262) -> (data=w267:variant, error out=w266:errorcluster)
                    n95 = stacked-sequence {
                      tunnel: w267 -> [w268]
                      tunnel: w266 -> [_]
                      frame #0 {
                        "Type 3" <- w268
                      }
                    }
                  }
                  frame Enabled {
                    n96 = call <vilib>:"Decode Application Message (Raw).vi"("PUBLISH"=w276, "Client in"=w277) -> ("error out"=→"error out 9":errorcluster, "Payload"=w273:u8[], "Client out"=w275:refnum<class "Client.lvclass">)  [unwired: 6 in, 1 out]
                    n97 = Byte Array To String(unsigned byte array=w273) -> (string=w272:string)
                    "K" <- w272
                    n98 = Fract/Exp String To Number(string=w272) -> (number=w270:dbl)  [unwired: 3 in, 1 out]
                    n99 = Greater?(x=w270, y="SET POINT K") -> (0:w269:bool)
                    n100 = case shown="True" w269 {
                      frame False {
                        # "Open"
                        n101 = local write "holding register value K"(u16 1 ("holding register value P")) -> ()
                        n102 = property on="Write Button" class="Bool (strict)"("Val(Sgnl)"=TRUE ("Value (Signaling)")) -> ()  [unwired: 2 in, 2 out]
                        "K" <- TRUE ("K")
                      }
                      frame True {
                        # "close"
                        n103 = local write "holding register value K"(u16 0 ("holding register value P")) -> ()
                        n104 = property on="Write Button" class="Bool (strict)"("Val(Sgnl)"=TRUE ("Value (Signaling)")) -> ()  [unwired: 2 in, 2 out]
                        n105 = local write "K"(FALSE ("K")) -> ()
                      }
                    }
                  }
                }
                n106 = feedback-in #1(w255) -> ()
              }
              frame "RawPayload" {
                n107 = call <vilib>:"Decode Application Message (Raw).vi"("error in (no error)"=w285, "PUBLISH"=w284, "Client in"=w289) -> ("error out"=w286:errorcluster, "Payload"=w287:u8[], "Client out"=w288:refnum<class "Client.lvclass">)  [unwired: 5 in, 1 out]
                n108 = stacked-sequence {
                  tunnel: w287 -> [_]
                  frame #0 {
                  }
                }
              }
              frame Default {
                # "Read Raw Payload"
                n109 = call <vilib>:"Read Payload.vi"("ControlPacket in"=w291) -> ("Payload"=→"Incoming Message":u8[])  [unwired: 9 in, 1 out]
              }
            }
          }
          event User Event {
            n110 = event-data() -> ()  [unwired: 1 in, 1 out]
          }
        }
        n111 = Compound Arithmetic op=OR(w125, w123) -> (w124:bool)
      }
    }
    frame True {
    }
  }
  n112 = call <vilib>:"Stop.vi"("error in (no error)"=w27, "MQTT_Base in"=w25) -> ("error out"=w26:errorcluster, "MQTT_Base out"=w24:refnum<class "Client.lvclass">)  [unwired: 7 in, 1 out]
  n113 = Unregister For Events(event registration refnum=w18) -> ()  [unwired: 1 in, 1 out]
  n114 = call <vilib>:"Destroy.vi"("error in (no error)"=w26, "MQTT_Base in"=w24) -> ("error out"=→"error out 2":errorcluster)  [unwired: 8 in, 1 out]
